vi "MVP02_P_CD backup.vi"() -> ()   [LabVIEW 2016]
uses:
  Custom Device/MVP02/MVP02 Custom Device.lvlib
panel:
  in  "error in (no error)":errorcluster
  out "error out":errorcluster
  in  "Repeticao":dbl format="%#_13g"
  in  "Caso Teste":dbl format="%#_13g"
  out "Gabarito":string
  out "String (OCR/OCV 1)":string
  out "Passed?":bool
  in  "milliseconds to wait":u32=100
  in  "stop":bool
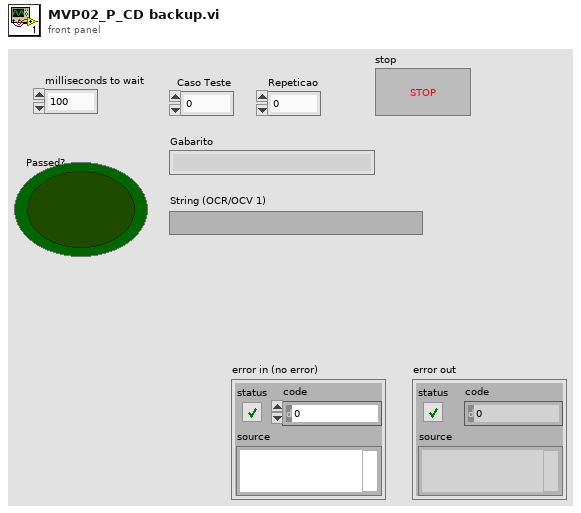
[diagram p1: front panel]
types:
  T1 = typedef "Vision Case.ctl" = enum16{"Espera", "OCR", "OCR2", "Outros"}
  T2 = typedef "IMAQ Image.ctl" = refnum<image>
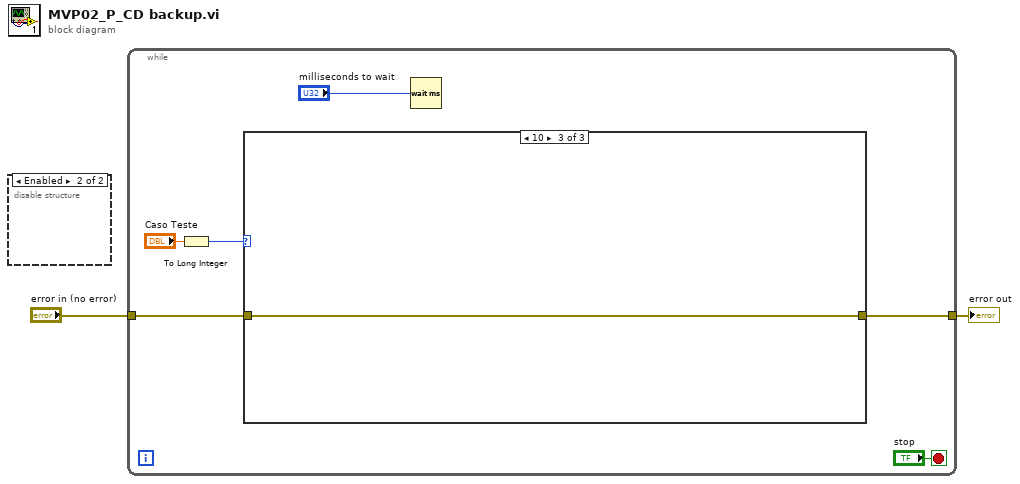
[diagram p0: block diagram]
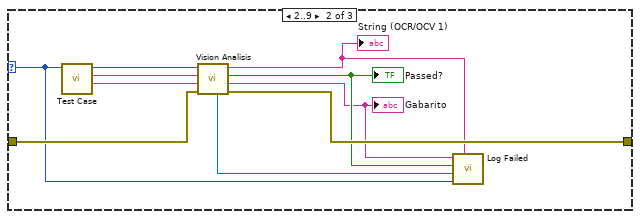
[diagram p3: hidden frame]
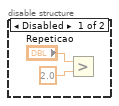
[diagram p4: hidden frame]
diagram:
  n1 = disable-structure shown="Enabled" {
    frame Disabled {
      n2 = Greater?(x="Repeticao", y=2.0) -> ()  [unwired: 1 out]
    }
    frame Enabled {
    }
  }
  n3 = while {
    tunnel: "error in (no error)" -> [w8]
    tunnel: [w7] -> w1
    stop <- "stop" stop-if-true
    n4 = To Long Integer(number="Caso Teste") -> (32bit integer=w5:i32)
    n5 = case shown="10" w5 {
      selector: w5 -> [_ w12 _]
      tunnel: w8 -> [w11 w21 w22]
      tunnel: [w11 w20 w22] -> w7
      frame 0, Default {
      }
      frame 2..9 {
        n6 = call "Test Case.vi"("Numeric"=w12) -> ("Linha 2"=w17:string, "Linha 1"=w18:string, "Image Case"=w19:T1)  [unwired: 8 in]
        n7 = call "Vision Analisis.vi"("error in"=w21, "Linha 2"=w17, "Linha 1"=w18, "Image Case"=w19) -> ("error out"=w20:errorcluster, "Gabarito"=w14:string, "Passed?"=w15:bool, "String (OCR/OCV 1)"=w13:string, "Image Out"=w16:T2)  [unwired: 3 in]
        "Passed?" <- w15
        "String (OCR/OCV 1)" <- w13
        "Gabarito" <- w14
        n8 = call "Log Failed.vi"("RESULTADO"=w13, "Case number"=w12, "Image In"=w16, "Boolean"=w15, "GABARITO"=w14) -> ()  [unwired: 7 in]
      }
      frame 10 {
      }
    }
    n9 = Wait (ms)(milliseconds to wait="milliseconds to wait") -> ()  [unwired: 1 out]
  }
  "error out" <- w1
